vi "Micron Optics sm130 Log Peak Wavelength.vi"() -> ()   [LabVIEW 2015]
doc: "Demonstrates peak wavelength and timestamp data logging. \n\n<b>Note:</b>\nThis example is made for the instrument without channel multiplexer. Modifications will have to be made for instruments with channel multiplexer."
uses:
  <vilib>/Utility/file.llb/Write To Spreadsheet File (string).vi
  <vilib>/Utility/file.llb/Write To Spreadsheet File (DBL).vi
  Micron Optics sm130.lvlib
panel:
  in  "Sample Rate (1000 Hz)":i32=1000
  in  "CH4 Sensor Number (1)":i32=1
  in  "CH3 Sensor Number (1)":i32=1
  in  "CH2 Sensor Number (1)":i32=1
  in  "CH1 Sensor Number (1)":i32=1
  out "Channel 4":dbl(graph)
  out "Channel 3":dbl(graph)
  out "Channel 2":dbl(graph)
  out "Channel 1":dbl(graph)
  in  "Stop":bool
  in  "VISA resource name":refnum<visa-resource-name>
  # "(c) 2009 - 2012 National Instruments.  ALL RIGHTS RESERVED."
  # "Sensor Number"
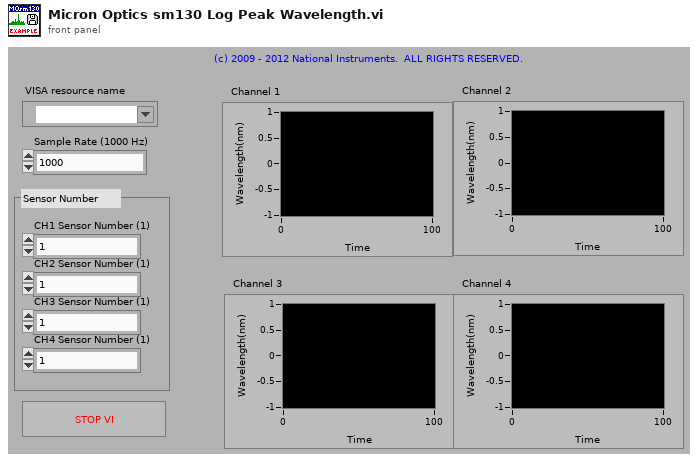
[diagram p1: front panel]
types:
  T1 = cluster{"Data Serial Number":u32, "Time Stamp":dbl, "Sub-Channel":u8}
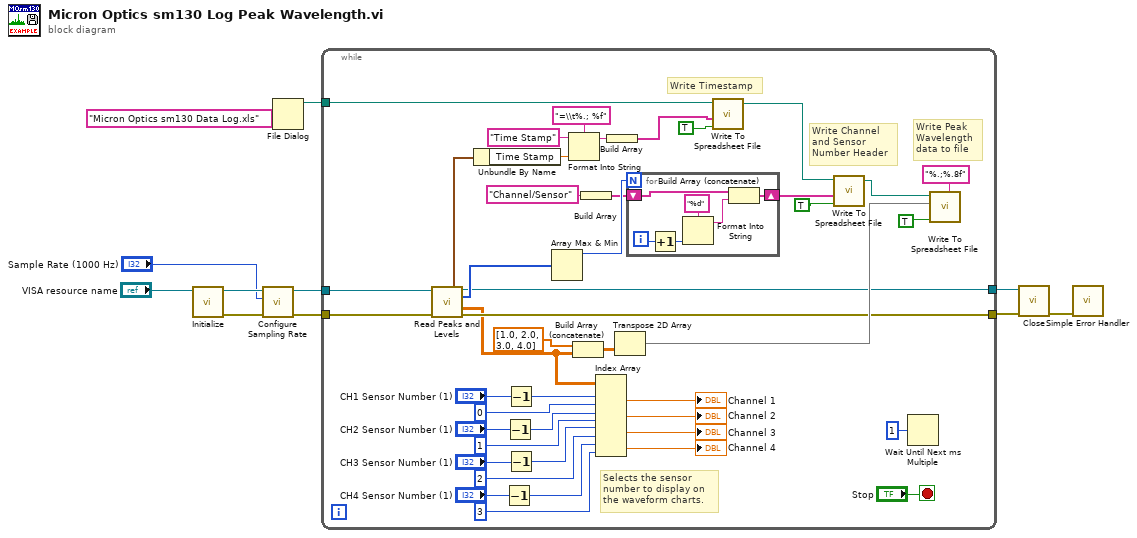
[diagram p0: block diagram]
diagram:
  n1 = call "Initialize.vi"("VISA resource name"="VISA resource name") -> ("error out"=w9:errorcluster, "VISA resource name out"=w10:refnum<visa-resource-name>)  [unwired: 9 in]
  n2 = call "Configure Sampling Rate.vi"("error in (no error)"=w9, "Sample Rate (1000 Hz)"="Sample Rate (1000 Hz)", "VISA resource name"=w10) -> ("error out"=w6:errorcluster, "VISA resource name out"=w7:refnum<visa-resource-name>)  [unwired: 7 in]
  n3 = File Dialog(9:"Micron Optics sm130 Data Log.xls" ("default name")) -> (3:w4:path)  [unwired: 6 in, 3 out]
  n4 = while {
    tunnel: w7 -> [w55]
    tunnel: w6 -> [w54]
    tunnel: w4 -> [w39]
    tunnel: [w31] -> w3
    tunnel: [w30] -> w2
    stop <- "Stop" stop-if-true
    # "Selects the sensor number to display on the waveform charts."
    # "Write Peak Wavelength data to file"
    # "Write Channel and Sensor Number Header"
    # "Write Timestamp"
    n5 = call "Read Peaks and Levels.vi"("VISA resource name"=w55, "error in (no error)"=w54) -> ("Data Status"=w44:T1, "VISA resource name out"=w31:refnum<visa-resource-name>, "Number of Sensors"=w53:u16[], "Peak Wavelengths (nm)"=w28:dbl[][], "error out"=w30:errorcluster)  [unwired: 8 in, 1 out]
    n6 = Unbundle By Name(w44) -> ("Time Stamp"=w36:dbl)
    n7 = Decrement(x="CH4 Sensor Number (1)") -> (x-1=w17:i32)
    n8 = Decrement(x="CH2 Sensor Number (1)") -> (x-1=w12:i32)
    n9 = Decrement(x="CH1 Sensor Number (1)") -> (x-1=w19:i32)
    n10 = Decrement(x="CH3 Sensor Number (1)") -> (x-1=w18:i32)
    n11 = Array Max & Min(array=w53) -> (max value=w51:u16)  [unwired: 3 out]
    n12 = Format Into String(format string="=\\t%.; %f", initial string="Time Stamp", w36) -> (resulting string=w33:string)  [unwired: 1 in, 1 out]
    n13 = Build Array (concatenate)(dbl[] [1.0, 2.0, 3.0, 4.0], w28) -> (w43:dbl[][])
    n14 = Build Array("Channel/Sensor" ("element")) -> (w48:string[])
    n15 = Index Array(array=w28, index (row) #1=w19, index (col) #1=0 ("disabled index (col)"), index (row) #2=w12, index (col) #2=1 ("index (col)"), index (row) #3=w18, index (col) #3=2 ("index (col)"), index (row) #4=w17, index (col) #4=3 ("index (col)")) -> (element #1=→"Channel 1":dbl, element #2=→"Channel 2":dbl, element #3=→"Channel 3":dbl, element #4=→"Channel 4":dbl)
    n16 = Build Array(w33) -> (w32:string[])
    n17 = Transpose 2D Array(2D array=w43) -> (transposed array=w40:dbl[][])
    n18 = for {
      N: w51 -> [_]
      shift-right: [w60] -> w50
      shift-left: w48 -> [w61]
      i -> [w58]
      n19 = Increment(x=w58) -> (x+1=w57:i32)
      n20 = Format Into String(format string="%d", w57) -> (resulting string=w59:string)  [unwired: 2 in, 1 out]
      n21 = Build Array (concatenate)(w61, w59) -> (w60:string[])
    }
    n22 = call-poly <vilib>:"Write To Spreadsheet File.vi"("append to file? (new file:F)"=TRUE, "1D data"=w32, "file path (dialog if empty)"=w39) -> ("new file path (Not A Path if cancelled)"=w38:path)  [unwired: 5 in]
    n23 = call-poly <vilib>:"Write To Spreadsheet File.vi"("append to file? (new file:F)"=TRUE, "1D data"=w50, "file path (dialog if empty)"=w38) -> ("new file path (Not A Path if cancelled)"=w46:path)  [unwired: 5 in]
    n24 = Wait Until Next ms Multiple(millisecond multiple=u32 1) -> ()  [unwired: 1 out]
    n25 = call-poly <vilib>:"Write To Spreadsheet File.vi"("format (%.3f)"="%.;%.8f", "append to file? (new file:F)"=TRUE, "2D data"=w40, "file path (dialog if empty)"=w46) -> ()  [unwired: 4 in, 1 out]
  }
  n26 = call "Close.vi"("error in (no error)"=w2, "VISA resource name"=w3) -> ("error out"=w1:errorcluster)  [unwired: 9 in]
  n27 = call <vilib>:"Simple Error Handler.vi"("error in (no error)"=w1) -> ()  [unwired: 4 in, 5 out]
